vi "Move.vi"(8 "error in (no error)":errorcluster, 9 "Absolute (T)":bool=TRUE, 10 "Point":refnum<class "Point.lvclass">, 11 "Point in":refnum<class "PointSpecialized.lvclass">) -> (0 "error out":errorcluster, 3 "Point out":refnum<class "PointSpecialized.lvclass">)   [LabVIEW 2021, in "Picture2D.lvlib" / "PointSpecialized.lvclass"]
uses:
  PointSpecialized.lvclass
  Point/Point.lvclass
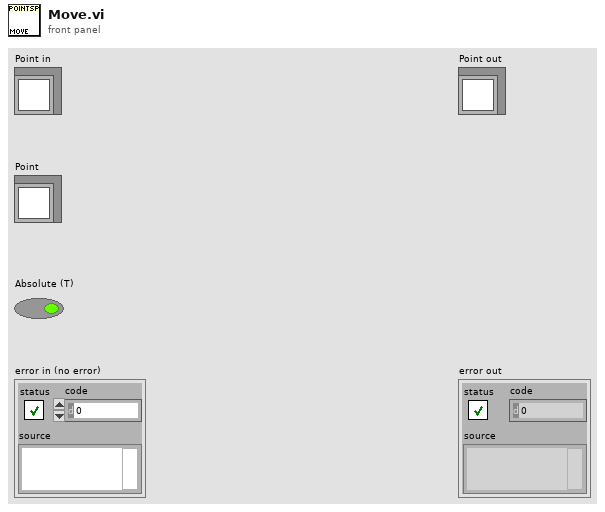
[diagram p1: front panel]
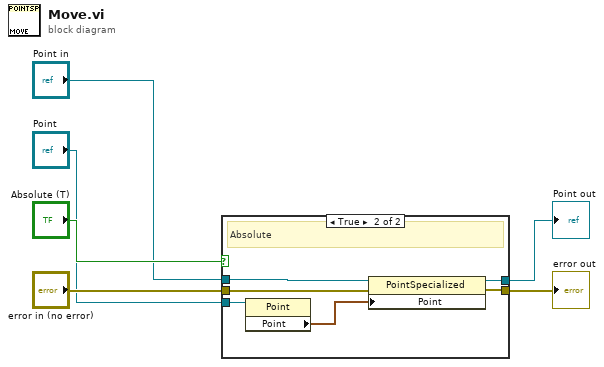
[diagram p0: block diagram]
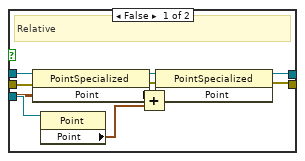
[diagram p2: hidden frame]
diagram:
  n1 = case shown="True" "Absolute (T)" {
    tunnel: "Point in" -> [w16 w22]
    tunnel: [w14 w21] -> w4
    tunnel: "Point" -> [w10 w18]
    tunnel: "error in (no error)" -> [w15 w20]
    tunnel: [w11 w19] -> w5
    frame False {
      # "Relative"
      n2 = property class="PointSpecialized"(reference=w16, error in=w15) -> (reference out=w13:refnum<class "PointSpecialized.lvclass">, error out=w12:errorcluster, "Point"=w9:cluster{"x":i16, "y":i16})
      n3 = property class="Point"(reference=w10) -> ("Point"=w8:cluster{"x":i16, "y":i16})  [unwired: 1 in, 2 out]
      n4 = Add(x=w9, y=w8) -> (x+y=w7:cluster{"x":i16, "y":i16})
      n5 = property class="PointSpecialized"(reference=w13, error in=w12, "Point"=w7) -> (reference out=w14:refnum<class "PointSpecialized.lvclass">, error out=w11:errorcluster)
    }
    frame True {
      # "Absolute"
      n6 = property class="Point"(reference=w18) -> ("Point"=w17:cluster{"x":i16, "y":i16})  [unwired: 1 in, 2 out]
      n7 = property class="PointSpecialized"(reference=w22, error in=w20, "Point"=w17) -> (reference out=w21:refnum<class "PointSpecialized.lvclass">, error out=w19:errorcluster)
    }
  }
  "error out" <- w5
  "Point out" <- w4
